vi "Shooter Motors.vi"(0 "State Control":enum16{"Open", "Run", "End"}(ring), 1 "Return":bool, 2 "Fire":bool, 3 "2 Ft":bool, 4 "4 ft":bool, 5 "Top Stop":bool, 6 "Encoder":dbl, 13 "Pickup in position":bool) -> (14 "Fully shot?":bool, 18 "Lower pickup":bool, 19 "Fully retracted?":bool)   [LabVIEW 2013]
uses:
  <vilib>/Rock Robotics/SystemInterfaces/DIO/FPGA_DIOPWMChannel.ctl
  <vilib>/Rock Robotics/WPI/MotorControl/WPI_MotorControlOpen Talon.vi
panel:
  in  "2 Feet":dbl=84.0
  in  "4 Feet":dbl=92.0 format="%#_13g"
  in  "Break":dbl format="%#_13g"
  in  "rest":dbl=0.1 format="%#_13g"
  in  "Break point":dbl=100.0 format="%#_13g"
  in  "Shoot":dbl=1.0 format="%#_13g"
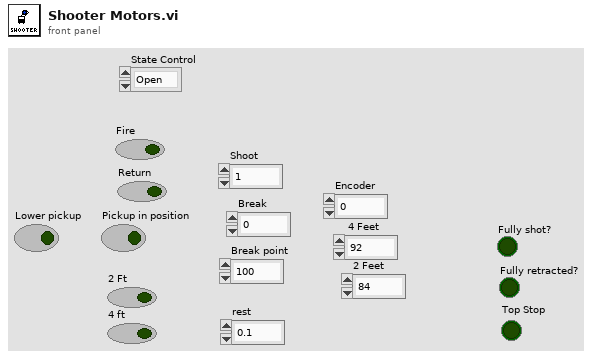
[diagram p1: front panel]
types:
  T1 = typedef "FPGA_DIOPWMChannel.ctl" = enum8{"PWM 1", "PWM 2", "PWM 3", "PWM 4", "PWM 5", "PWM 6", "PWM 7", "PWM 8", "PWM 9", "PWM 10", "Invalid"}
  T2 = typedef "WPI_MotorControlDeviceRef.ctl" = cluster{"DeviceStatus":errorcluster, "Type":enum16{"PWM", "CAN"}, "PWM":cluster{"Digital Module":T3, "PWM Channel":T1, "DeadBand":T4}, "CAN":cluster{"Device Number":u8, "Control Mode":T5, "Semaphore":T6, "Max Vout":dbl}, "Invert":bool, "TransformRef":T7, "InvTransformRef":T7}
  T3 = typedef "FPGA_TypedefDigitalModule.ctl" = enum16{"Digital Module 1", "Digital Module 2"}
  T4 = typedef "WPI_PWMDeadband.ctl" = cluster{"Name":string, "maxPositivePwm":i32, "minPositivePwm":i32, "centerPwm":i32, "maxNegativePwm":i32, "minNegativePwm":i32, "angularRange":u16}
  T5 = typedef "WPI_CANJaguar_ControlMode.ctl" = enum8{"Percent VBus", "Current", "Speed", "Position", "Voltage"}
  T6 = typedef "Semaphore RefNum" = refnum<k1>
  T7 = typedef "WPI_PWMTransform_ConPane.ctl" = refnum<vi>
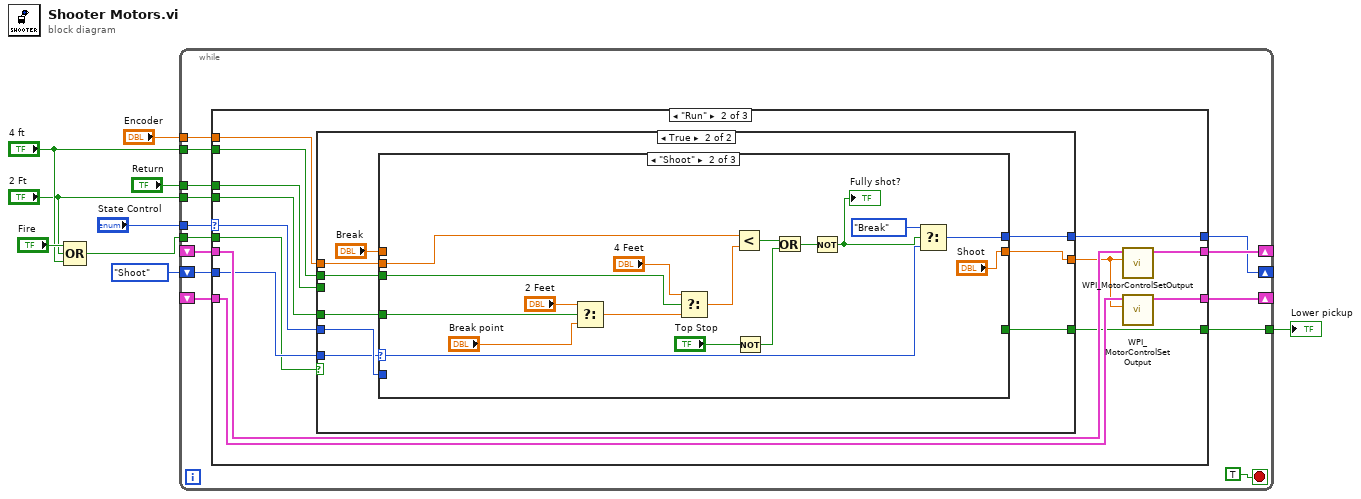
[diagram p0: block diagram]
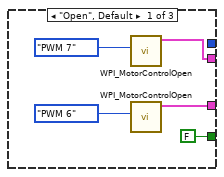
[diagram p2: hidden frame]
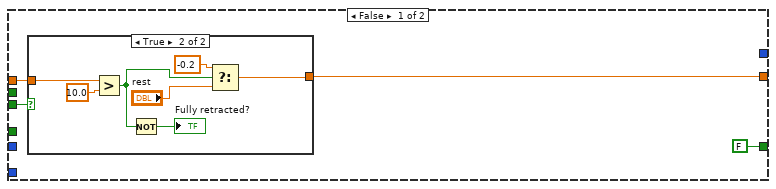
[diagram p3: hidden frame]
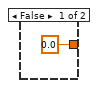
[diagram p4: hidden frame]
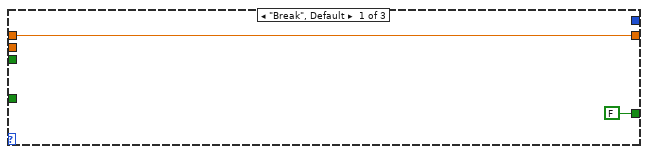
[diagram p5: hidden frame]
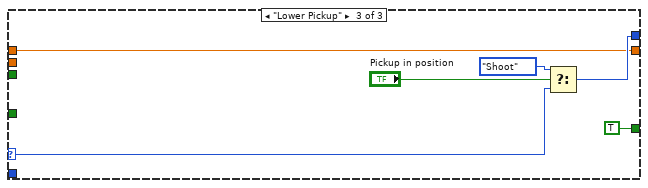
[diagram p6: hidden frame]
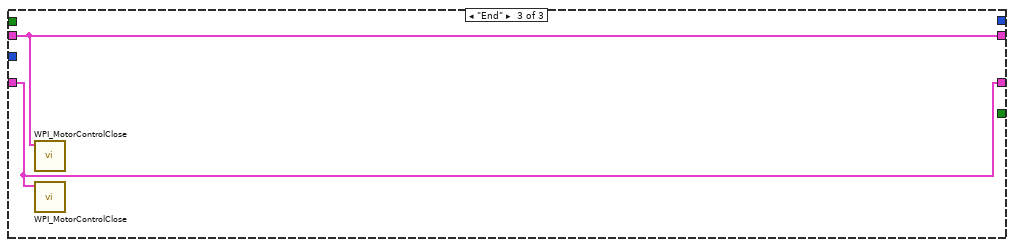
[diagram p7: hidden frame]
diagram:
  n1 = Compound Arithmetic op=OR("Fire", "2 Ft", "4 ft") -> (w3:bool)
  n2 = while {
    shift-right: [w23] -> _
    shift-left: _ -> [w22]
    tunnel: "State Control" -> [w21]
    shift-right: [w19] -> _
    shift-left: _ -> [w18]
    tunnel: w3 -> [w17]
    tunnel: "Return" -> [w16]
    tunnel: "Encoder" -> [w15]
    shift-right: [w14] -> _
    shift-left: enum16{"Break", "Shoot", "Lower Pickup"}."Shoot" ("Shooting State") -> [w13]
    tunnel: [w12] -> w5
    tunnel: "4 ft" -> [w11]
    tunnel: "2 Ft" -> [w10]
    stop <- TRUE stop-if-true
    n3 = case shown="\"Run\"" w21 {
      selector: w21 -> [_ w35 _]
      tunnel: [w26 w39 w90] -> w23
      tunnel: w22 -> [_ w41 w90]
      tunnel: [w25 w38 w89] -> w19
      tunnel: w18 -> [_ w42 w89]
      tunnel: w17 -> [_ w31 _]
      tunnel: w16 -> [_ w37 _]
      tunnel: w15 -> [_ w36 _]
      tunnel: [_ w34 _] -> w14
      tunnel: w13 -> [_ w33 _]
      tunnel: [FALSE w32 _] -> w12
      tunnel: w11 -> [_ w30 _]
      tunnel: w10 -> [_ w29 _]
      frame "Open", Default {
        n4 = call-poly <vilib>:"WPI_MotorControlOpen.vi"("PWM Channel"=FPGA_DIOPWMChannel."PWM 7" ("PWMChannel")) -> ("MotorControlDeviceRef"=w25:T2)  [unwired: 9 in, 1 out]
        n5 = call-poly <vilib>:"WPI_MotorControlOpen.vi"("PWM Channel"=FPGA_DIOPWMChannel."PWM 6" ("PWMChannel")) -> ("MotorControlDeviceRef"=w26:T2)  [unwired: 9 in, 1 out]
      }
      frame "Run" {
        n6 = case shown="True" w31 {
          tunnel: [w45 w59] -> w40
          tunnel: w37 -> [w46 _]
          tunnel: w36 -> [w44 w60]
          tunnel: w35 -> [_ w63]
          tunnel: [_ w62] -> w34
          tunnel: w33 -> [_ w61]
          tunnel: [FALSE w57] -> w32
          tunnel: w30 -> [_ w56]
          tunnel: w29 -> [_ w55]
          frame False {
            n7 = case shown="True" w46 {
              tunnel: [0.0 w50] -> w45
              tunnel: w44 -> [_ w54]
              frame False {
              }
              frame True {
                n8 = Greater?(x=w54, y=10.0) -> (0:w49:bool)
                n9 = Not(x=w49) -> (.not. x?=→"Fully retracted?":bool)
                n10 = Select(t=-0.2, s=w49, f="rest") -> (s? t:f=w50:dbl)
              }
            }
          }
          frame True {
            n11 = case shown="\"Shoot\"" w61 {
              selector: w61 -> [_ w76 w87]
              tunnel: w63 -> [_ _ _]
              tunnel: [_ w74 w86] -> w62
              tunnel: w60 -> [_ w78 _]
              tunnel: [w65 "Shoot" w85] -> w59
              tunnel: "Break" -> [w65 _ w85]
              tunnel: [FALSE _ TRUE] -> w57
              tunnel: w56 -> [_ w69 _]
              tunnel: w55 -> [_ w68 _]
              frame "Break", Default {
              }
              frame "Shoot" {
                n12 = Select(t="2 Feet", s=w68, f="Break point") -> (s? t:f=w71:dbl)
                n13 = Select(t="4 Feet", s=w69, f=w71) -> (s? t:f=w72:dbl)
                n14 = Less?(x=w78, y=w72) -> (x < y?=w79:bool)
                n15 = Not(x="Top Stop") -> (.not. x?=w81:bool)
                n16 = Or(x=w79, y=w81) -> (x .or. y?=w80:bool)
                n17 = Not(x=w80) -> (.not. x?=w75:bool)
                "Fully shot?" <- w75
                n18 = Select(t=enum16{"Break", "Shoot", "Lower Pickup"}."Break" ("Shooting State"), s=w75, f=w76) -> (s? t:f=w74:enum16{"Break", "Shoot", "Lower Pickup"})
              }
              frame "Lower Pickup" {
                n19 = Select(t=enum16{"Break", "Shoot", "Lower Pickup"}."Shoot" ("Shooting State"), s="Pickup in position", f=w87) -> (s? t:f=w86:enum16{"Break", "Shoot", "Lower Pickup"})
              }
            }
          }
        }
        n20 = call <vilib>:"WPI_MotorControlSetOutput.vi"("Output"=w40, "MotorControlDevRef"=w42) -> ("MotorControlDevRef"=w38:T2)  [unwired: 7 in, 2 out]
        n21 = call <vilib>:"WPI_MotorControlSetOutput.vi"("Output"=w40, "MotorControlDevRef"=w41) -> ("MotorControlDevRef"=w39:T2)  [unwired: 7 in, 2 out]
      }
      frame "End" {
        n22 = call <vilib>:"WPI_MotorControlClose.vi"("MotorControlDevRef"=w89) -> ()  [unwired: 10 in, 1 out]
        n23 = call <vilib>:"WPI_MotorControlClose.vi"("MotorControlDevRef"=w90) -> ()  [unwired: 10 in, 1 out]
      }
    }
  }
  "Lower pickup" <- w5
